vi "Write Mfg Peltier Test Timestamp.vi"(8 "error in":errorcluster, 11 "Time Stamp":timestamp) -> (0 "error out":errorcluster)   [LabVIEW 2015]
uses:
  CAN Communication/Peltier/Peltier.lvclass
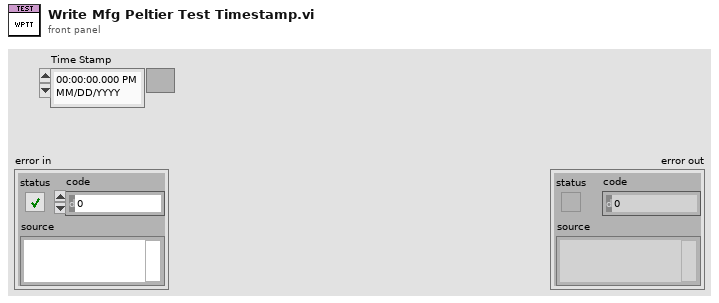
[diagram p1: front panel]
types:
  T1 = typedef "Peltier.lvclass/Session Handle.ctl" = refnum<data-value>
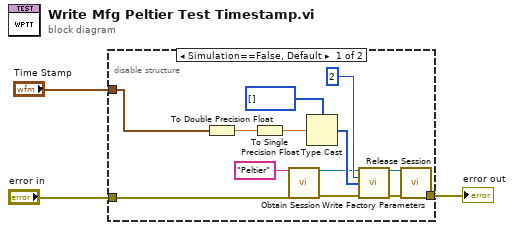
[diagram p0: block diagram]
diagram:
  n1 = disable-structure shown="Simulation==False, Default" {
    disable-tunnel: "error in" -> [w16 w17]
    disable-tunnel: [w15 w17] -> w2
    disable-tunnel: "Time Stamp" -> [w4 _]
    frame condition #0 (active) {
      n2 = To Double Precision Float(number=w4) -> (double precision float=w14:dbl)
      n3 = To Single Precision Float(number=w14) -> (single precision float=w10:sgl)
      n4 = call "Obtain Session.vi"("Session  Name ()"="Peltier", "error in (no error)"=w16) -> ("Session Handle"=w5:T1, "error out"=w12:errorcluster)  [unwired: 12 in]
      n5 = Type Cast(type=u8[] [] ("Bytes to Write"), x=w10) -> (*(type *) &x=w8:u8[])
      n6 = call "Write Factory Parameters.vi"("Session Handle in"=w5, "Address"=u16 2, "Bytes to Write"=w8, "error in (no error)"=w12) -> ("Session Handle out"=w6:T1, "error out"=w7:errorcluster)  [unwired: 10 in]
      n7 = call "Release Session.vi"("Session Handle"=w6, "error in (no error)"=w7) -> ("error out"=w15:errorcluster)  [unwired: 13 in]
    }
    frame condition #1 {
    }
  }
  "error out" <- w2
